vi "Write.vi"(8 "error in (no error)":errorcluster, 10 "Data":u64, 11 "CIFTag in":refnum<class "CIFTagU64.lvclass">) -> (0 "error out":errorcluster, 1 "timed out?":bool, 3 "CIFTag out":refnum<class "CIFTagU64.lvclass">)   [LabVIEW 2021, in "CIFTagU64.lvclass"]
uses:
  CIFTagU64.lvclass
  D:/dev/CIF-LVCore/src/Channels/CIFTag/CIFTag/CIFTag.lvclass
  CIFTag/CIFTag.lvclass/CIFTag.ctl
  CIFTagU64.lvclass/CIFTagU64.ctl
  e6e5dc56-0fe0-434b-816e-55c2e61471c2.vi
  e6e5dc56-0fe0-434b-816e-55c2e61471c2.vi/4bc1c15b-36ab-481f-b8dd-c64075ce723a.vi
  e6e5dc56-0fe0-434b-816e-55c2e61471c2.vi/d83cb72b-7713-41fc-a3d1-682de79cf574.vi
  <vilib>/CIFChannels/SubVIs/Get dll Path.vi
  CIFTag/CIFTag.lvclass
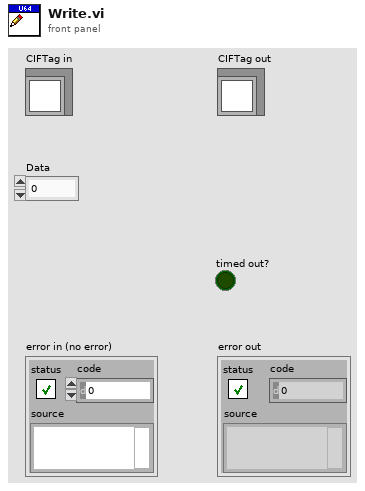
[diagram p1: front panel]
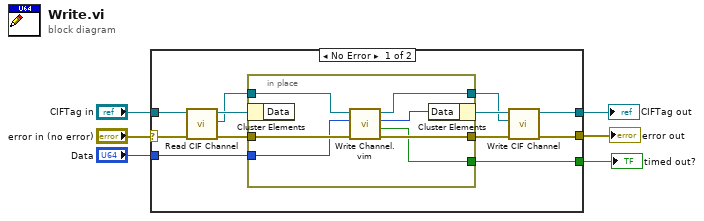
[diagram p0: block diagram]
diagram:
  n1 = case shown="No Error" "error in (no error)" {
    selector: "error in (no error)" -> [w15 w27]
    tunnel: [w9 w27] -> w5
    tunnel: [w11 w26] -> w3
    tunnel: "CIFTag in" -> [w16 w26]
    tunnel: "Data" -> [w18 _]
    tunnel: [w17 _] -> w1
    frame No Error {
      n2 = call "Read CIF Channel.vi"("error in (no error)"=w15, "CIFTag in"=w16) -> ("error out"=w13:errorcluster, "CIF Channel"=w8:refnum<k21>, "CIFTag out"=w14:refnum<class "CIFTagU64.lvclass">)  [unwired: 7 in]
      n3 = in-place {
        in-place-border: w13 -> [w25]
        in-place-border: [w24] -> w10
        in-place-border: w18 -> [w22]
        in-place-border: [w23] -> w17
        in-place-border: w8 -> [w20]
        in-place-border: [w19] -> w7
        n4 = in-place-cluster #1(w14) -> ()  [unwired: 1 out]
        n5 = call "Write Channel.vim"("error in"=w25, "Data in"=w22, "CIF Channel in"=w20) -> ("error out"=w24:errorcluster, "Timed out?"=w23:bool, "Data out"=w21:u64, "CIF Channel out"=w19:refnum<k21>)  [unwired: 5 in]
        n6 = in-place-cluster #1("Data"=w21) -> (w12:refnum<class "CIFTagU64.lvclass">)
      }
      n7 = call "Write CIF Channel.vi"("error in (no error)"=w10, "CIF Channel"=w7, "CIFTag in"=w12) -> ("error out"=w9:errorcluster, "CIFTag out"=w11:refnum<class "CIFTagU64.lvclass">)  [unwired: 7 in]
    }
    frame Error {
    }
  }
  "error out" <- w5
  "CIFTag out" <- w3
  "timed out?" <- w1
